vi "Delay.vi"(1 "error in (no error)":errorcluster, 2 "Wait (s)":i32) -> (0 "error out":errorcluster)   [LabVIEW 2020]
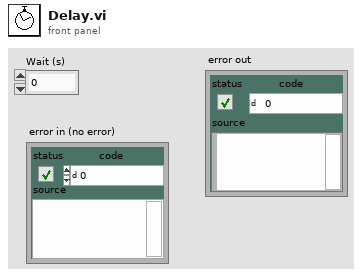
[diagram p1: front panel]
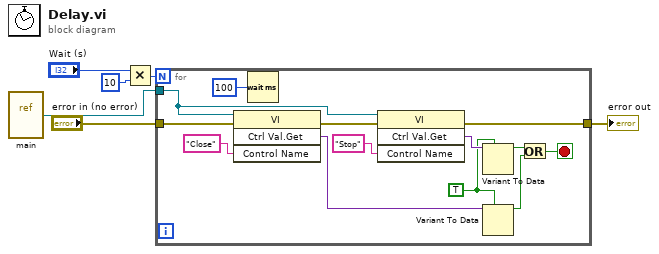
[diagram p0: block diagram]
diagram:
  n1 = vi-ref "main.vi"() -> (w3:refnum<vi>)
  n2 = Multiply(x="Wait (s)", y=10) -> (x*y=w4:i32)
  n3 = for {
    N: w4 -> [_]
    tunnel: w3 -> [w10]
    tunnel: "error in (no error)" -> [w11]
    tunnel: [w7] -> w1
    stop <- w15 stop-if-true
    w16 = TRUE
    n4 = invoke class="VI" method="Ctrl Val.Get"(reference=w10, error in=w11, "Control Name"="Close") -> (error out=w8:errorcluster, "Get Control Value Variant"=w17:variant)  [unwired: 1 in, 2 out]
    n5 = Wait (ms)(milliseconds to wait=u32 100) -> ()  [unwired: 1 out]
    n6 = invoke class="VI" method="Ctrl Val.Get"(reference=w10, error in=w8, "Control Name"="Stop") -> (error out=w7:errorcluster, "Get Control Value Variant"=w18:variant)  [unwired: 1 in, 2 out]
    n7 = Variant To Data(type=w16, Variant=w18) -> (data=w14:bool)  [unwired: 1 in, 1 out]
    n8 = Variant To Data(type=w16, Variant=w17) -> (data=w13:bool)  [unwired: 1 in, 1 out]
    n9 = Or(x=w14, y=w13) -> (x .or. y?=w15:bool)
  }
  "error out" <- w1
